vi "H5Pget_cache.vi"(8 "error in (no error)":errorcluster, 11 "HDF5 Property List Ref":T1) -> (0 "error out":errorcluster, 1 "rdcc_nbytes":u64, 2 "rdcc_nelmts":u64, 3 "HDF5 Property List Ref out":T1, 4 "rdcc_w0":dbl, 5 "mdc_nelmts":i32)   [LabVIEW 2017]
doc: "Queries the raw data chunk cache parameters."
uses:
  <vilib>/UPVI/lvhdf5/library.llb/HDF5 Ref.ctl
  <vilib>/UPVI/lvhdf5/hdf5.dll
panel:
  # "LVHDF5 Toolkit\nCopyright (c) 2005-2013 by Jason D. Sommerville\nCopyright (c) 2014 by UPVI, LLC.\n\nThis use and distribution of this file is governed by the terms found in \nLICENSE.txt distributed with this toolkit and installed at\n <user.lib>\\_lvhdf5\\LICENSE.txt"
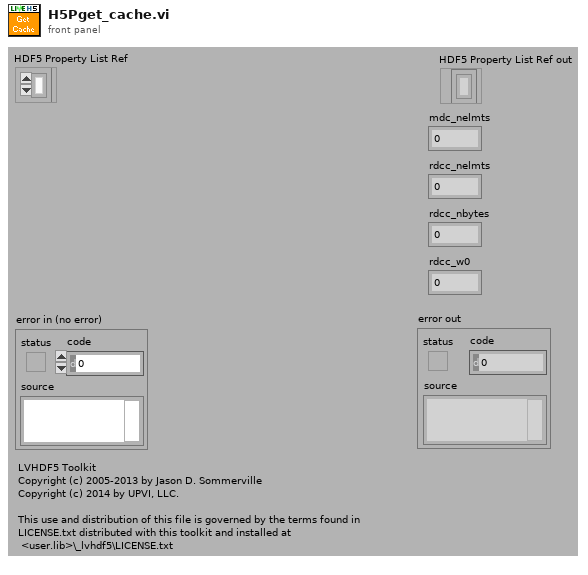
[diagram p1: front panel]
types:
  T1 = typedef "HDF5 Ref.ctl" = refnum<k1>
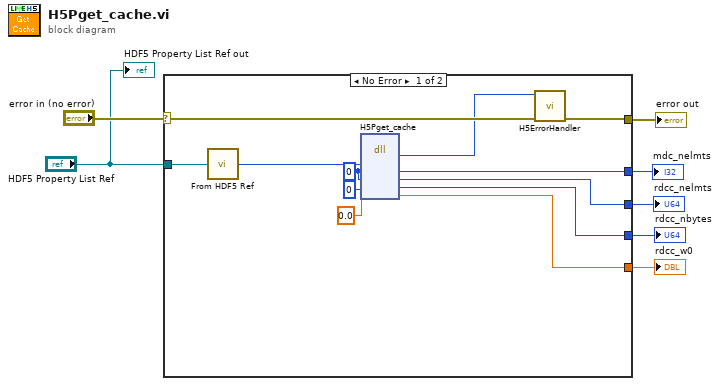
[diagram p0: block diagram]
diagram:
  n1 = case shown="No Error" "error in (no error)" {
    selector: "error in (no error)" -> [w19 w20]
    tunnel: [w18 w20] -> w6
    tunnel: "HDF5 Property List Ref" -> [w17 _]
    tunnel: [w11 _] -> w4
    tunnel: [w10 _] -> w3
    tunnel: [w9 _] -> w2
    tunnel: [w8 _] -> w1
    frame No Error {
      w14 = 0 ("mdc_nelmts")
      n2 = call <vilib>:"From HDF5 Ref.vi"("HDF5 Ref"=w17) -> ("I32"=w16:i32)
      n3 = dll-call lib="C:/Program Files/National Instruments/LabVIEW 2017/vi.lib/UPVI/lvhdf5/hdf5.dll" fn="H5Pget_cache"("plist_id"=w16, "mdc_nelmts"=w14, "rdcc_nelmts"=w14, "rdcc_nbytes"=u32 0, "rdcc_w0"=0.0) -> ("return type"=w15:i32, "mdc_nelmts"=w11:i32, "rdcc_nelmts"=w10:u64, "rdcc_nbytes"=w9:u64, "rdcc_w0"=w8:dbl)  [unwired: 4 in, 2 out]
      n4 = call <vilib>:"H5ErrorHandler.vi"("error in (no error)"=w19, "herr_t"=w15) -> ("error out"=w18:errorcluster)  [unwired: 3 in, 4 out]
    }
    frame Error {
    }
  }
  "error out" <- w6
  "mdc_nelmts" <- w4
  "rdcc_nelmts" <- w3
  "rdcc_nbytes" <- w2
  "rdcc_w0" <- w1
  "HDF5 Property List Ref out" <- "HDF5 Property List Ref"
